vi "Write MAIN printer IP Value.vi"(8 "error in (no error)":errorcluster, 10 "printer IP value":string, 11 "Domino Laser module Class in":refnum<class "Domino Laser module Class.lvclass">) -> (0 "error out":errorcluster, 3 "Domino Laser module Class out":refnum<class "Domino Laser module Class.lvclass">)   [LabVIEW 2015, in "Domino LM.lvlib" / "Domino Laser module Class.lvclass"]
uses:
  CTRLS/Domino Laser module Class.lvclass
  CTRLS/Domino Laser module Class.lvclass/Domino Laser module Class.ctl
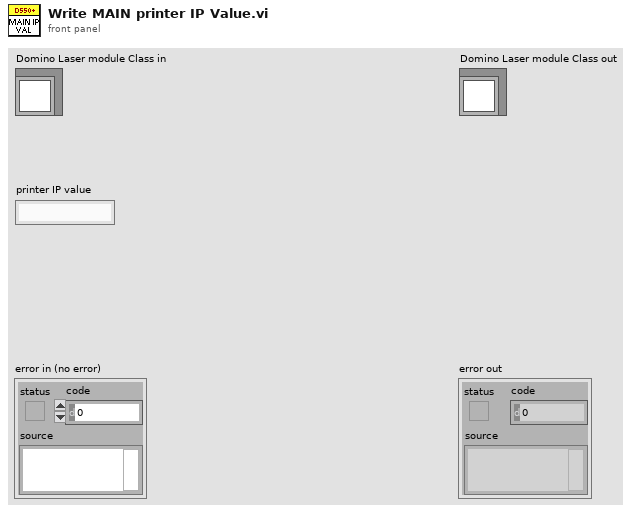
[diagram p1: front panel]
types:
  T1 = cluster{"Printer  IP":string, "Printer B IP":string, "Delay SSCC Print [S]":string}
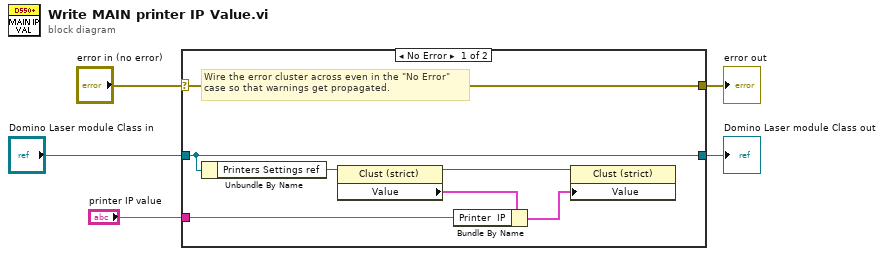
[diagram p0: block diagram]
diagram:
  n1 = case shown="No Error" "error in (no error)" {
    selector: "error in (no error)" -> [w12 w14]
    tunnel: [w12 w14] -> w4
    tunnel: [w11 w13] -> w2
    tunnel: "Domino Laser module Class in" -> [w11 w13]
    tunnel: "printer IP value" -> [w7 _]
    frame No Error {
      # "Wire the error cluster across even in the \"No Error\"\ncase so that warnings get propagated."
      n2 = Unbundle By Name(w11) -> ("Printers Settings ref"=w10:refnum<vi>)
      n3 = property class="Clust (strict)"(reference=w10) -> (reference out=w6:refnum<vi>, "Value"=w9:T1)  [unwired: 1 in, 1 out]
      n4 = Bundle By Name(cluster=w9, "Printer  IP"=w7) -> (w8:T1)
      n5 = property class="Clust (strict)"(reference=w6, "Value"=w8) -> ()  [unwired: 1 in, 2 out]
    }
    frame Error {
    }
  }
  "error out" <- w4
  "Domino Laser module Class out" <- w2
